vi "Conditionally Serialiaze.vi"(8 "error in (no error)":errorcluster, 11 "Device Item Ref in":T1 format="%.0x") -> (0 "error out":errorcluster)   [LabVIEW 2011]
uses:
  <vilib>/NI Veristand/Custom Device API/Custom Device Item Ref.ctl
  <vilib>/NI Veristand/Custom Device API/Get Item Property (Path).vi
  Controls and Global/Global.vi
  <vilib>/NI Veristand/Custom Device API/NI VeriStand - Add Custom Device Dependencies.vi
  <vilib>/NI Veristand/Custom Device API/NI VeriStand - Reset Custom Device Dependencies.vi
  <vilib>/NI Veristand/Custom Device API/Custom Device API.lvlib
  AIT 1553 Custom Device.lvlib
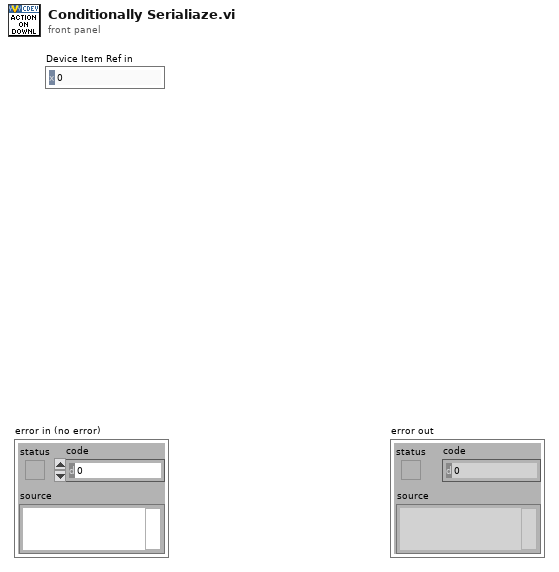
[diagram p1: front panel]
types:
  T1 = typedef "Custom Device API.lvlib/Custom Device Item Ref.ctl" = u64
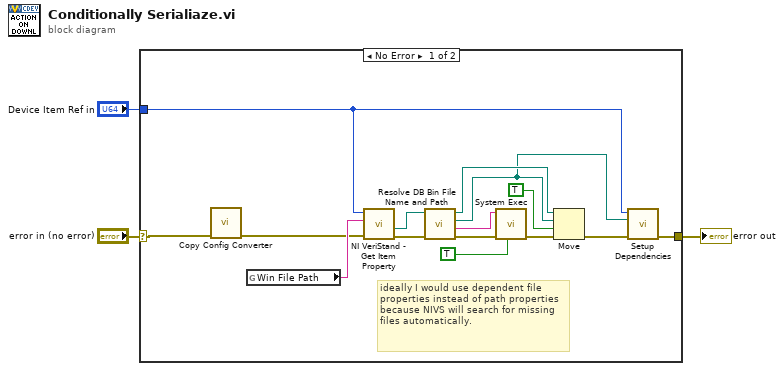
[diagram p0: block diagram]
diagram:
  n1 = case shown="No Error" "error in (no error)" {
    selector: "error in (no error)" -> [w5 w19]
    tunnel: [w17 w19] -> w2
    tunnel: "Device Item Ref in" -> [w16 _]
    frame No Error {
      # "ideally I would use dependent file properties instead of path properties because NIVS will search for missing files automatically."
      n2 = call "Copy Config Converter.vi"("error in (no error)"=w5) -> ("error out"=w4:errorcluster)  [unwired: 10 in]
      n3 = global read "Global.vi" "Win File Path"() -> (w18:string)
      n4 = call-poly <vilib>:"NI VeriStand - Get Item Property.vi"("error in (no error)"=w4, "Property Name"=w18, "Item Ref in"=w16) -> ("error out"=w13:errorcluster, "Value"=w9:path)  [unwired: 5 in, 2 out]
      n5 = call "Resolve DB Bin File Name and Path.vi"("error in"=w13, "DB XML File"=w9) -> ("error out"=w12:errorcluster, "SysExec"=w8:string, "Destination File"=w6:path, "Converted File"=w7:path)  [unwired: 6 in]
      n6 = call <vilib>:"System Exec.vi"("run minimized? (F)"=TRUE, "error in (no error)"=w12, "command line"=w8) -> ("error out"=w11:errorcluster)  [unwired: 5 in, 3 out]
      n7 = Move(source path=w7, error in=w11, 9:TRUE ("overwrite (F)"), 10:w6) -> (error out=w10:errorcluster)  [unwired: 1 in, 2 out]
      n8 = call "Setup Dependencies.vi"("error in (no error)"=w10, "Windows Bin File"=w6, "Item Ref in"=w16) -> ("error out"=w17:errorcluster)  [unwired: 8 in]
    }
    frame Error {
    }
  }
  "error out" <- w2
